vi "Get Children.vi"(8 "error in (no error)":errorcluster, 11 "Data Item in":refnum<class "Data Item.lvclass">) -> (0 "error out":errorcluster, 2 "Children":refnum<class "Data Item.lvclass">[](array[class]), 3 "Data Item out":refnum<class "Data Item.lvclass">)   [LabVIEW 2018, in "VILab.lvlib" / "Data Item.lvclass"]
uses:
  Data Item.lvclass
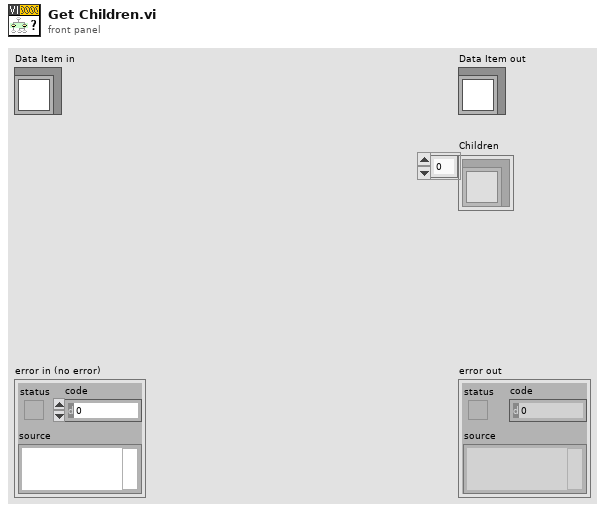
[diagram p1: front panel]
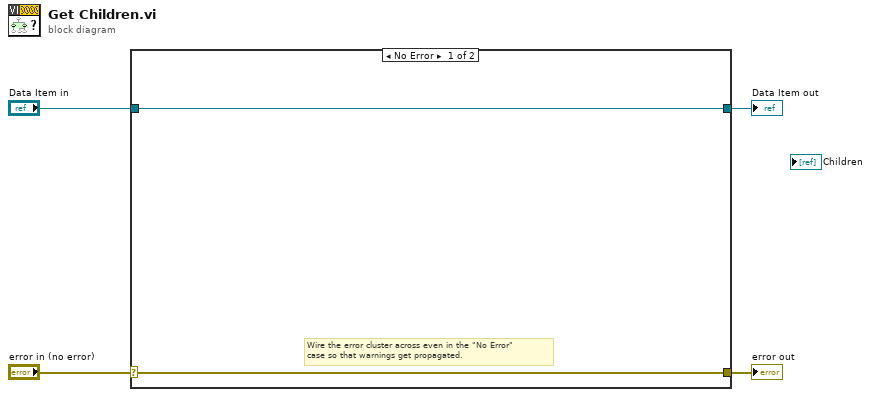
[diagram p0: block diagram]
diagram:
  n1 = case shown="No Error" "error in (no error)" {
    selector: "error in (no error)" -> [w5 w8]
    tunnel: [w5 w8] -> w3
    tunnel: [w6 w7] -> w1
    tunnel: "Data Item in" -> [w6 w7]
    frame No Error {
      # "Wire the error cluster across even in the \"No Error\"\ncase so that warnings get propagated."
    }
    frame Error {
    }
  }
  "error out" <- w3
  "Data Item out" <- w1
